vi "Combine Results.vi"(8 "error in (no error)":errorcluster, 11 "Combined Measurement in":refnum<class "Combined Measurement.lvclass">) -> (0 "error out":errorcluster, 3 "Combined Measurement out":refnum<class "Combined Measurement.lvclass">)   [LabVIEW 2021, in "Combined Measurement.lvclass"]
uses:
  Combined Measurement.lvclass
  C:/GitHub/LabActor/Worker/Worker Actor/Worker Actor.lvclass
  Worker/Worker Actor/Worker Actor.lvclass/Worker Actor.ctl
  NHMFL_Core/Libraries/Instruments/Results/Acquired Result/Acquired Result.lvclass/Acquired Result.ctl
  NHMFL_Core/Libraries/Instruments/Results/Acquired Result/Write Group.vi
  Worker/Worker Actor/Read Cycle count.vi
  Measurements/Response Synchronizer/Response Synchronizer.lvclass
  NHMFL_Core/Libraries/Instruments/Results/Combined Result/Combined Result.lvclass
  Combined Measurement.lvclass/Combined Measurement.ctl
  NHMFL_Core/Libraries/Instruments/Results/Acquired Result/Acquired Result.lvclass
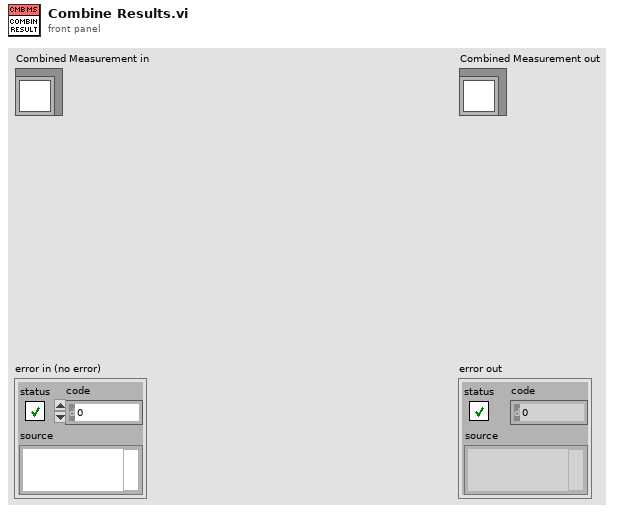
[diagram p1: front panel]
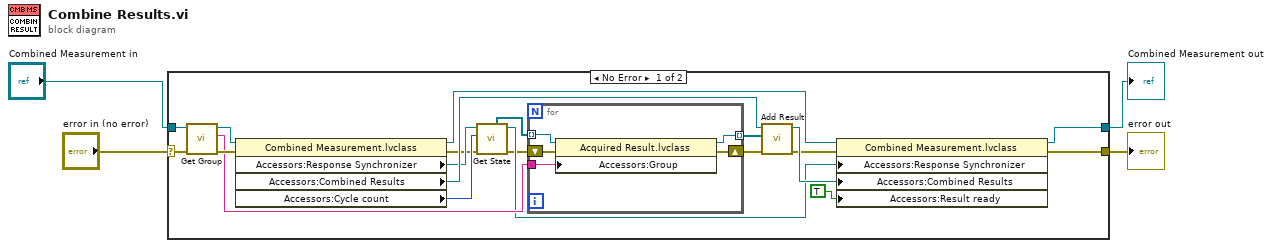
[diagram p0: block diagram]
diagram:
  n1 = case shown="No Error" "error in (no error)" {
    selector: "error in (no error)" -> [w16 w30]
    tunnel: [w6 w31] -> w2
    tunnel: "Combined Measurement in" -> [w17 w31]
    tunnel: [w5 w30] -> w1
    frame No Error {
      n2 = call-dynamic "Get Group.vi"("error in (no error)"=w16, "Combined Measurement in"=w17) -> ("error out"=w20:errorcluster, "Group"=w18:string, "Combined Measurement out"=w19:refnum<class "Combined Measurement.lvclass">)  [unwired: 7 in]
      n3 = property class="Combined Measurement.lvclass"(reference=w19, error in=w20) -> (reference out=w24:refnum<class "Combined Measurement.lvclass">, error out=w9:errorcluster, "Accessors:Response Synchronizer"=w11:refnum<class "Response Synchronizer.lvclass">, "Accessors:Combined Results"=w14:refnum<class "Combined Result.lvclass">, "Accessors:Cycle count"=w12:i32)
      n4 = call-dynamic "Get State.vi"("error in (no error)"=w9, "Cycle count"=w12, "Response Synchronizer in"=w11) -> ("error out"=w8:errorcluster, "Response Synchronizer out"=w10:refnum<class "Response Synchronizer.lvclass">, "Results"=w7:refnum<class "Acquired Result.lvclass">[])  [unwired: 3 in, 3 out]
      n5 = for {
        tunnel: w7 -> [w27] mode=indexing
        tunnel: w18 -> [w29]
        tunnel: [w26] -> w22 mode=indexing
        shift-right: [w25] -> w21
        shift-left: w8 -> [w28]
        n6 = property class="Acquired Result.lvclass"(reference=w27, error in=w28, "Accessors:Group"=w29) -> (reference out=w26:refnum<class "Acquired Result.lvclass">, error out=w25:errorcluster)
      }
      n7 = call-dynamic "Add Result.vi"("error in (no error)"=w21, "Results to add"=w22, "Combined Result in"=w14) -> ("error out"=w13:errorcluster, "Combined Result out"=w23:refnum<class "Combined Result.lvclass">)  [unwired: 7 in]
      n8 = property class="Combined Measurement.lvclass"(reference=w24, error in=w13, "Accessors:Response Synchronizer"=w10, "Accessors:Combined Results"=w23, "Accessors:Result ready"=TRUE ("Result ready")) -> (reference out=w6:refnum<class "Combined Measurement.lvclass">, error out=w5:errorcluster)
    }
    frame Error {
    }
  }
  "error out" <- w1
  "Combined Measurement out" <- w2
